vi "Detect_circles_detectors.vi"(5 "Detectors":T4(array[cluster]), 6 "Match_score":dbl, 7 "Circle Descriptor":cluster{"Min Radius":dbl, "Max Radius":dbl}, 8 "error in (no error)":errorcluster, 9 "Curve Parameters":T3 {"Max Endpoint Gap" min=0; "Col Search Step Size" min=1 max=255 step=1; "Row Search Step Size" min=1 max=255 step=1; "Min Length" min=0; "Edge Filter Size" items=["Fine", "Normal", "Controur Tracing"]; "Edge Threshold" min=1 max=65535 step=1; "Extraction Mode" items=["Normal", "Uniform Regions"]}, 10 "Match Options":T1 {"Range Settings"."Match Constraints" items=["Rotation Angle (degrees)", "Scale Factor (%)", "Occlusion (%)"]}, 11 "Refnum in":T5) -> (0 "error out":errorcluster, 3 "Array":sgl[][](array[numeric]))   [LabVIEW 2020]
uses:
  <vilib>/vision/Image Controls.llb/IMAQ Image.ctl
  <vilib>/vision/Pattern Matching.llb/IMAQ Curve Parameters.ctl
  <vilib>/vision/Shape Detection.llb/ShapeDetectionMatchOptions.ctl
  <vilib>/vision/Pattern Matching.llb/IMAQ Match Range Setting.ctl
  <vilib>/vision/NI_Vision_Development_Module.lvlib
panel:
  # "Range"
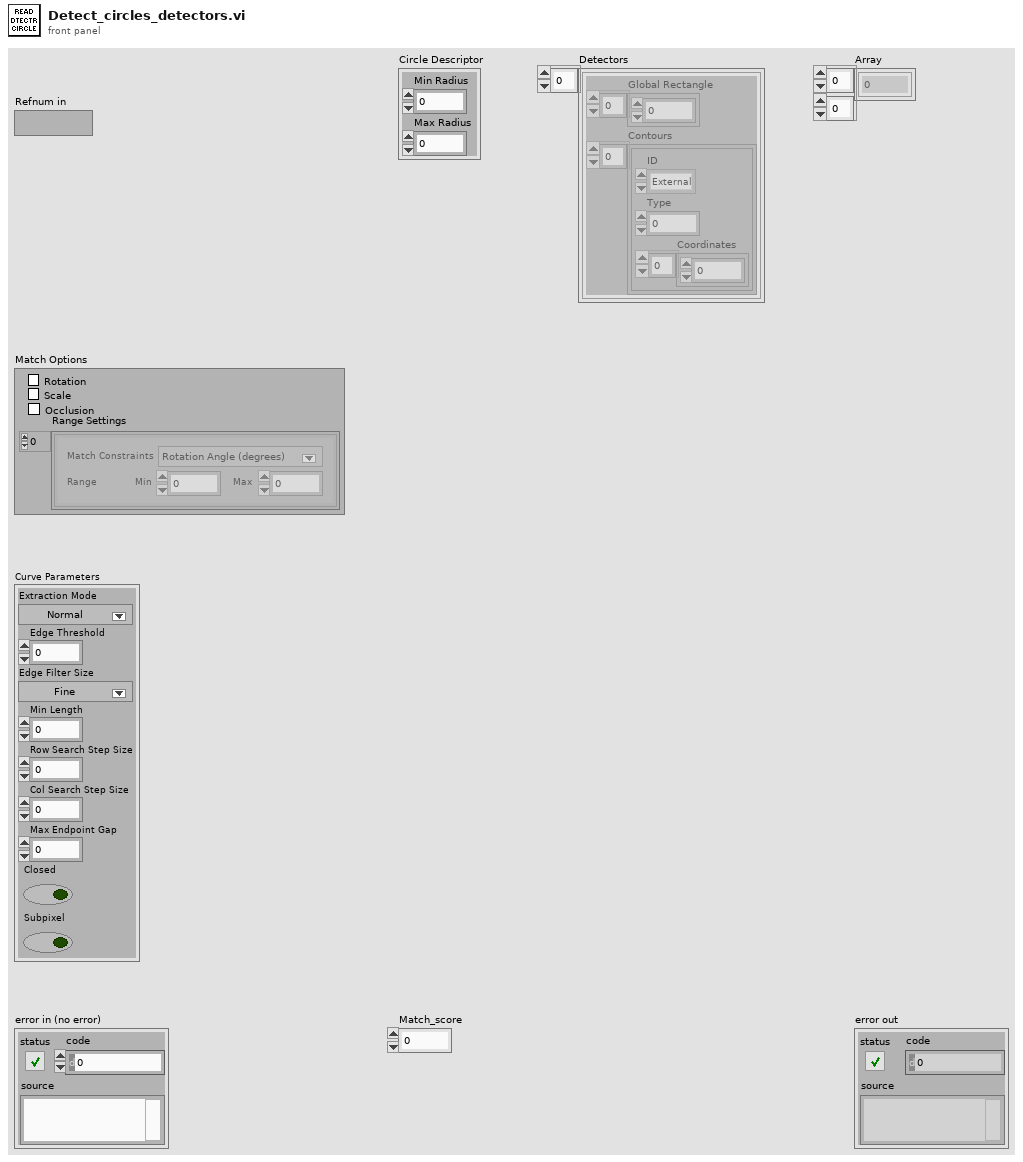
[diagram p1: front panel]
types:
  T1 = typedef "ShapeDetectionMatchOptions.ctl" = cluster{"Rotation":bool, "Scale":bool, "Occlusion":bool, "Range Settings":T2[]}
  T2 = typedef "IMAQ Match Range Setting.ctl" = cluster{"Match Constraints":u32, "Min":dbl, "Max":dbl}
  T3 = typedef "IMAQ Curve Parameters.ctl" = cluster{"Extraction Mode":u32, "Edge Threshold":i32, "Edge Filter Size":u32, "Min Length":i32, "Row Search Step Size":i32, "Col Search Step Size":i32, "Max Endpoint Gap":i32, "Closed":bool, "Subpixel":bool}
  T4 = cluster{"Global Rectangle":i32[], "Contours":cluster{"ID":enum32{"External", "Internal"}, "Type":u32, "Coordinates":i32[]}[]}[]
  T5 = typedef "IMAQ Image.ctl" = refnum<image>
  T6 = cluster{"Position":cluster{"X":sgl, "Y":sgl}, "Radius":dbl, "Score":dbl}[]
  T7 = cluster{"Position":cluster{"X":sgl, "Y":sgl}, "Radius":dbl, "Score":dbl}
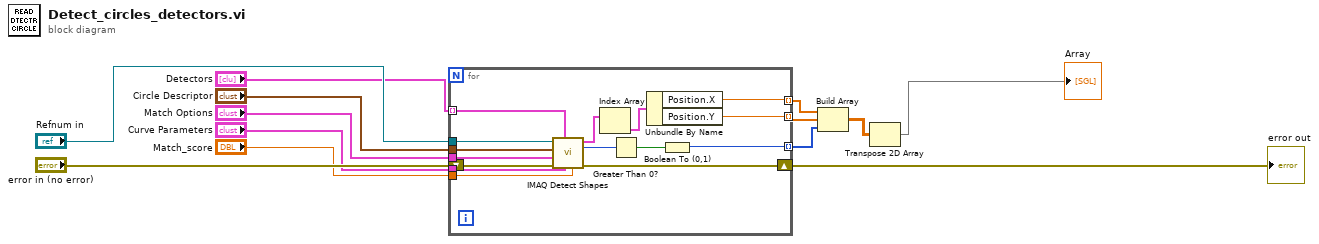
[diagram p0: block diagram]
diagram:
  n1 = for {
    tunnel: "Refnum in" -> [w28]
    tunnel: "Circle Descriptor" -> [w25]
    tunnel: "Match Options" -> [w24]
    tunnel: "Curve Parameters" -> [w23]
    tunnel: "Match_score" -> [w22]
    shift-right: [w26] -> w1
    shift-left: "error in (no error)" -> [w27]
    tunnel: "Detectors" -> [w21] mode=indexing
    tunnel: [w17] -> w9 mode=indexing
    tunnel: [w16] -> w7 mode=indexing
    tunnel: [w15] -> w8 mode=indexing
    n2 = call-poly "IMAQ Detect Shapes"("Minimum match score"=w22, "Curve Parameters"=w23, "ROI Descriptor"=w21, "error in (no error)"=w27, "Match Options"=w24, "Circle Descriptor"=w25, "Image"=w28) -> ("error out"=w26:errorcluster, "Number of Matches Returned"=w19:i32, "Circles"=w20:T6)  [unwired: 2 in]
    n3 = Index Array(array=w20) -> (element=w14:T7)  [unwired: 1 in]
    n4 = Greater Than 0?(x=w19) -> (x > 0?=w18:bool)
    n5 = Unbundle By Name(w14) -> ("Position.X"=w16:sgl, "Position.Y"=w15:sgl)
    n6 = Boolean To (0,1)(Boolean=w18) -> (0, 1=w17:i16)
  }
  "error out" <- w1
  n7 = Build Array(w7, w8, w9) -> (w10:sgl[][])
  n8 = Transpose 2D Array(2D array=w10) -> (transposed array=→"Array":sgl[][])
